vi "CPP-5168PuffReleaseAnalysisDevelopment.vi"() -> (5 "Plug in titles":string[](array[string]), 7 "Plug in values":string[](array[string]))   [LabVIEW 2012]
uses:
  Controls/Post_Process.ctl
  Globals/Meas_global.vi
  <vilib>/measure/mascope.llb/Transition Measurements 1 chan.vi
  <vilib>/Analysis/baseanly.llb/Quick Scale 1D.vi
  <vilib>/Analysis/baseanly.llb/Mean (DBL).vi
  <vilib>/measure/NI_MAPro.lvlib
  <vilib>/Analysis/NI_AALBase.lvlib
panel:
  in  "CPP-5168-FIDandPressure-Jan2013.vi Running Too?":bool=TRUE
  out "SampleLength":i32
  in  "MedianFilter(points)":i32=100
  in  "PufferCard":tag="PXI1Slot2"
  out "FFID1 2":cluster{dbl, dbl, dbl[]}[](graph)=[{3.0, 0.004, [20831.978051375965, 20830.73969787809, 20829.501417993935, 20828.26321171912, 20827.025079049276, 20825.787019980024, 20824.54903450699, 20823.311122625797, 20822.073284332073, 20820.83551962144, 20819.597828489525, 20818.360210931958, 20817.12266694436, 20815.885196522362, 20814.64779966159, 20813.410476357665, 20812.173226606224, 20810.936050402892, 20809.69894774329, 20808.461918623056, 20807.224963037814, 20805.98808098319, 20804.751272454818, 20803.51453744832, 20802.27787595934, 20801.041287983488, 20799.804773516407, 20798.56833255373, 20797.331965091074, 20796.09567112408, 20794.85945064838, 20793.623303659602, 20792.387230153374, 20791.151230125335, 20789.915303571113, 20788.679450486343, 20787.44367086665, 20786.20796470768, 20784.97233200505, 20783.736772754408, 20782.50128695138, 20781.265874591605, 20780.03053567071, 20778.795270184335, 20777.560078128114, 20776.32495949768, 20775.089914288666, 20773.854942496713, 20772.620044117455, 20771.38521914653, 20770.150467579566, 20768.915789412207, 20767.681184640092, 20766.44665325885, 20765.212195264125, 20763.977810651548, 20762.743499416763, 20761.509261555406, 20760.275097063113, 20759.041005935527, 20757.806988168282, 20756.573043757024, 20755.339172697382, 20754.105374985003, 20752.87165061553, 20751.637999584593, 20750.40442188784, 20749.17091752091, 20747.937486479444, 20746.704128759084, 20745.470844355466, 20744.237633264238, 20743.004495481044, 20741.771431001514, 20740.538439821306, 20739.30552193605, 20738.0726773414, 20736.839906032987, 20735.607208006462, 20734.37458325747, 20733.142031781652, 20731.909553574653, 20730.67714863212, 20729.444816949694, 20728.21255852302, 20726.980373347746, 20725.748261419518, 20724.516222733975, 20723.284257286774, 20722.052365073556, 20720.820546089963, 20719.588800331647, 20718.357127794257, 20717.125528473436, 20715.894002364836, 20714.662549464098, 20713.431169766878, 20712.19986326882, 20710.968629965573, 20709.737469852786, 20708.50638292611, 20707.27536918119, 20706.04442861368, 20704.81356121923, 20703.582766993495, 20702.35204593211, 20701.12139803074, 20699.890823285034, 20698.660321690637, 20697.429893243203, 20696.199537938388, 20694.96925577184, 20693.739046739214, 20692.50891083616, 20691.27884805833, 20690.04885840138, 20688.81894186096, 20687.58909843273, 20686.35932811234, 20685.12963089544, 20683.90000677769, 20682.670455754742, 20681.440977822254, 20680.211572975877, 20678.98224121127, 20677.75298252408, 20676.52379690998, 20675.29468436461, 20674.065644883634, 20672.836678462707, 20671.607785097483, 20670.378964783624, 20669.150217516788, 20667.921543292632, 20666.69294210681, 20665.464413954982, 20664.235958832807, 20663.007576735945, 20661.779267660055, 20660.551031600793, 20659.322868553823, 20658.094778514802, 20656.866761479392, 20655.63881744325, 20654.41094640204, 20653.183148351418, 20651.955423287054, 20650.727771204598, 20649.50019209972, 20648.272685968084, 20647.045252805343, 20645.817892607163, 20644.59060536921, 20643.363391087143, 20642.136249756626, 20640.90918137332, 20639.6821859329, 20638.455263431013, 20637.228413863337, 20636.001637225527, 20634.774933513254, 20633.548302722185, 20632.321744847977, 20631.095259886297, 20629.868847832815, 20628.642508683195, 20627.416242433108, 20626.19004907821, 20624.963928614176, 20623.737881036668, 20622.51190634136, 20621.286004523914, 20620.060175579998, 20618.83441950528, 20617.608736295435, 20616.383125946122, 20615.157588453014, 20613.93212381178, 20612.70673201809, 20611.481413067617, 20610.25616695602, 20609.03099367898, 20607.805893232162, 20606.58086561124, 20605.355910811882, 20604.131028829757, 20602.906219660545, 20601.681483299908, 20600.45681974352, 20599.232228987057, 20598.00771102619, 20596.78326585659, 20595.55889347393, 20594.33459387389, 20593.110367052133, 20591.886213004338, 20590.662131726178, 20589.438123213327, 20588.214187461464, 20586.990324466256, 20585.766534223385, 20584.54281672852, 20583.31917197734, 20582.095599965523, 20580.87210068874, 20579.648674142667, 20578.425320322985, 20577.202039225373, 20575.9788308455, 20574.75569517905, 20573.532632221697, 20572.309641969117, 20571.086724416993, 20569.863879561, 20568.64110739682, 20567.418407920126, 20566.195781126604, 20564.973227011928, 20563.750745571782, 20562.52833680184, 20561.306000697787, 20560.083737255303, 20558.861546470067, 20557.63942833776, 20556.417382854062, 20555.19541001466, 20553.97350981523, 20552.751682251455, 20551.52992731902, 20550.308245013606, 20549.086635330892, 20547.865098266564, 20546.643633816308, 20545.422241975804, 20544.200922740736, 20542.979676106785, 20541.758502069642, 20540.53740062499, 20539.31637176851, 20538.09541549589, 20536.87453180281, 20535.653720684964, 20534.43298213803, 20533.2123161577, 20531.991722739658, 20530.77120187959, 20529.55075357318, 20528.33037781612, 20527.110074604097, 20525.8898439328, 20524.66968579791, 20523.44960019512, 20522.229587120117, 20521.009646568586, 20519.789778536226, 20518.569983018715, 20517.35026001175, 20516.13060951102, 20514.91103151221, 20513.69152601101, 20512.472093003118, 20511.25273248422, 20510.033444450004, 20508.814228896164, 20507.595085818393, 20506.376015212383, 20505.15701707382, 20503.938091398402, 20502.71923818182, 20501.500457419766, 20500.281749107933, 20499.063113242017, 20497.844549817703, 20496.626058830694, 20495.407640276684, 20494.18929415136, 20492.971020450423, 20491.752819169564, 20490.534690304477, 20489.31663385086, 20488.09864980441, 20486.880738160817, 20485.662898915787, 20484.445132065004, 20483.227437604175, 20482.00981552899, 20480.792265835145, 20479.57478851835, 20478.357383574283, 20477.140050998656, 20475.922790787165, 20474.705602935504, 20473.488487439376, 20472.271444294474, 20471.054473496504, 20469.83757504116, 20468.620748924146, 20467.40399514116, 20466.187313687904, 20464.97070456007, 20463.75416775337, 20462.537703263497, 20461.321311086158, 20460.10499121705, 20458.888743651874, 20457.672568386337, 20456.456465416137, 20455.240434736974, 20454.024476344555, 20452.808590234585, 20451.592776402762, 20450.377034844794, 20449.161365556378, 20447.945768533224, 20446.73024377104, 20445.51479126552, 20444.29941101237, 20443.084103007306, 20441.86886724602, 20440.653703724227, 20439.43861243763, 20438.22359338193, 20437.008646552837, 20435.79377194606, 20434.578969557304, 20433.364239382274, 20432.14958141668, 20430.934995656226, 20429.720482096625, 20428.506040733584, 20427.291671562805, 20426.077374580003, 20424.863149780886, 20423.64899716116, 20422.434916716535, 20421.220908442723, 20420.00697233543, 20418.79310839037, 20417.579316603256, 20416.365596969794, 20415.15194948569, 20413.938374146666, 20412.724870948423, 20411.51143988668, 20410.298080957145, 20409.084794155533, 20407.871579477553, 20406.658436918922, 20405.44536647535, 20404.232368142548, 20403.019441916233, 20401.806587792114, 20400.59380576591, 20399.381095833338, 20398.168457990105, 20396.955892231927, 20395.74339855452, 20394.530976953603, 20393.318627424884, 20392.106349964088, 20390.894144566922, 20389.682011229102, 20388.469949946357, 20387.25796071439, 20386.04604352892, 20384.83419838567, 20383.622425280355, 20382.410724208694, 20381.1990951664, 20379.9875381492, 20378.776053152804, 20377.56464017293, 20376.353299205304, 20375.14203024564, 20373.93083328966, 20372.719708333087, 20371.508655371632, 20370.297674401023, 20369.086765416978, 20367.87592841522, 20366.665163391463, 20365.454470341436, 20364.243849260853, 20363.03330014545, 20361.82282299093, 20360.61241779303, 20359.402084547462, 20358.19182324996, 20356.981633896237, 20355.771516482022, 20354.56147100304, 20353.35149745501, 20352.141595833655, 20350.931766134705, 20349.72200835388, 20348.512322486906, 20347.302708529514, 20346.09316647742, 20344.883696326353, 20343.67429807204, 20342.464971710207, 20341.25571723658, 20340.046534646888, 20338.837423936853, 20337.62838510221, 20336.419418138674, 20335.21052304198, 20334.001699807857, 20332.792948432034, 20331.584268910236, 20330.37566123819, 20329.16712541163, 20327.958661426284, 20326.75026927788, 20325.541948962145, 20324.333700474814, 20323.125523811614, 20321.917418968278, 20320.709385940532, 20319.501424724112, 20318.293535314748, 20317.08571770817, 20315.87797190011, 20314.6702978863, 20313.46269566247, 20312.25516522436, 20311.047706567697, 20309.840319688214, 20308.63300458164, 20307.425761243718, 20306.218589670178, 20305.011489856748, 20303.80446179917, 20302.597505493177, 20301.3906209345, 20300.18380811888, 20298.977067042044, 20297.770397699736, 20296.56380008769, 20295.357274201633, 20294.150820037314, 20292.94443759046, 20291.738126856813, 20290.531887832112, 20289.325720512086, 20288.11962489248, 20286.913600969026, 20285.70764873747, 20284.50176819354, 20283.295959332983, 20282.09022215153, 20280.884556644934, 20279.678962808917, 20278.47344063923, 20277.26799013161, 20276.062611281795, 20274.857304085526, 20273.652068538548, 20272.446904636596, 20271.241812375414, 20270.036791750743, 20268.83184275832, 20267.626965393894, 20266.422159653204, 20265.217425531995, 20264.012763026003, 20262.80817213098, 20261.60365284266, 20260.399205156788, 20259.194829069114, 20257.990524575376, 20256.78629167132, 20255.582130352694, 20254.378040615233, 20253.174022454692, 20251.97007586681, 20250.766200847338, 20249.562397392012, 20248.358665496587, 20247.155005156805, 20245.951416368414, 20244.74789912716, 20243.54445342879, 20242.34107926905, 20241.13777664369, 20239.934545548454, 20238.731385979092, 20237.528297931352, 20236.325281400987, 20235.122336383734, 20233.919462875354, 20232.71666087159, 20231.51393036819, 20230.311271360908, 20229.108683845494, 20227.906167817695, 20226.703723273262, 20225.50135020795, 20224.299048617504, 20223.096818497677]}, ...(15 in all)]
  out "Valve":cluster{dbl, dbl, dbl[]}(graph)
  out "ValveShutAt":dbl format="%.2f"
  out "FFID2":T1(graph)
  out "Current Block No":i32
  out "FFID1":cluster{dbl, dbl, dbl[]}[](graph)
  out "SourceOffIndex":i32
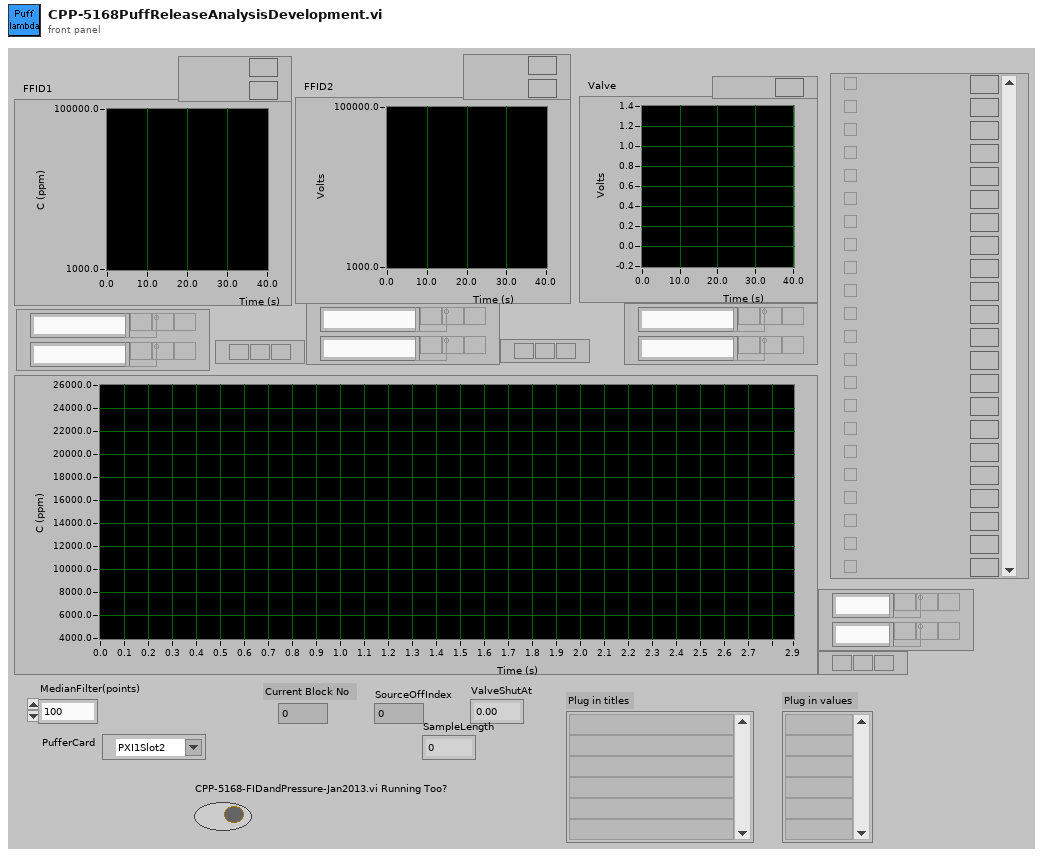
[diagram p1: front panel]
types:
  T1 = cluster{dbl, "SamplingRate":dbl, "Best Exponential Fit":dbl[]}[]
  T2 = typedef "Time_Trace_Cluster.ctl" = cluster{"Weighting":dbl[], "Time (s)":dbl[], "Voltage":dbl[], "Eng Values":dbl[]}
  T3 = typedef "Post_Process.ctl" = enum16{"Take New Data", "Post Process Raw Data File"}
  T4 = cluster{"start time":dbl, "end time":dbl, "ref levels":cluster{"high ref level":dbl, "mid ref level":dbl, "low ref level":dbl, "ref units":u16}}
  T5 = cluster{"x*y":dbl, "SamplingRate":dbl, "Filtered X":dbl[]}
  T6 = cluster{"x*y":dbl, "SamplingRate":dbl, "Filtered X":dbl[]}[]
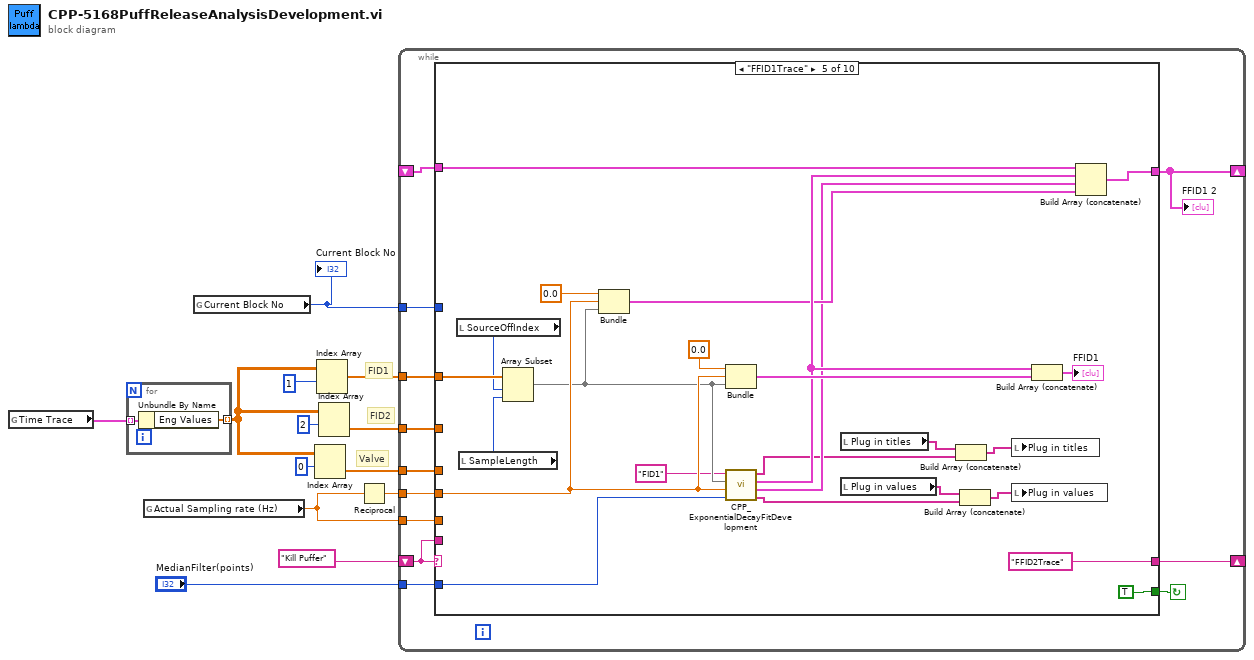
[diagram p0: block diagram]
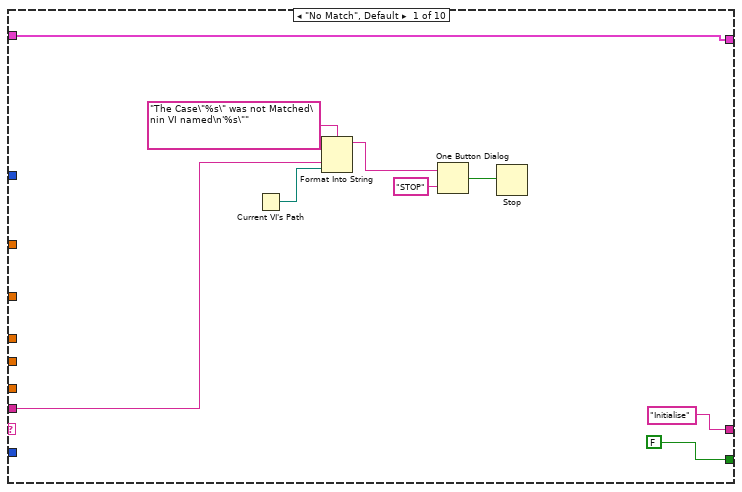
[diagram p2: hidden frame]
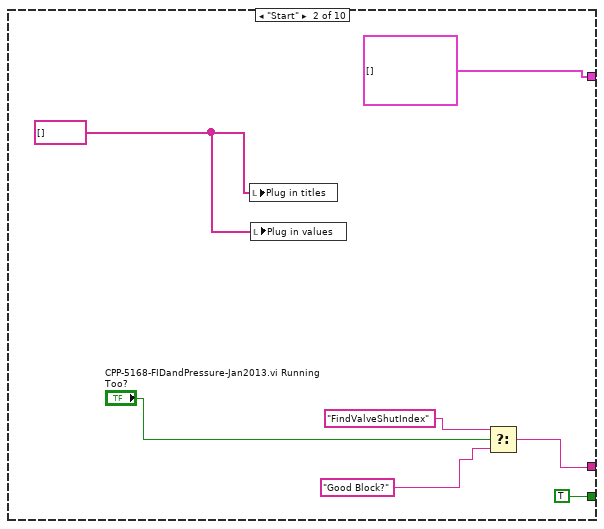
[diagram p3: hidden frame]
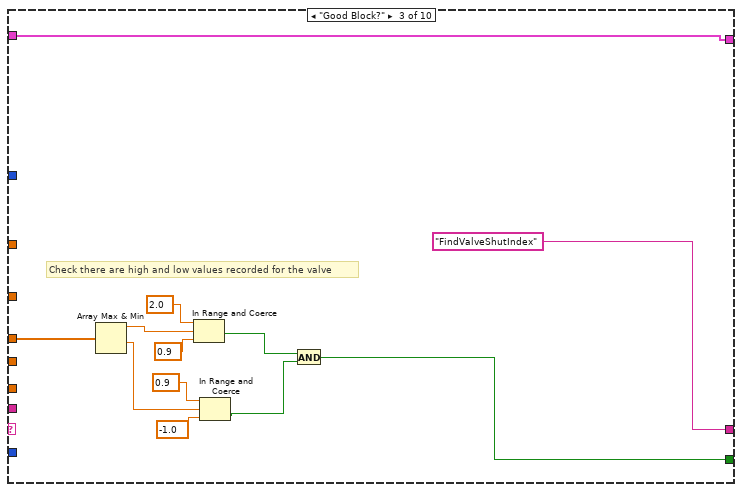
[diagram p4: hidden frame]
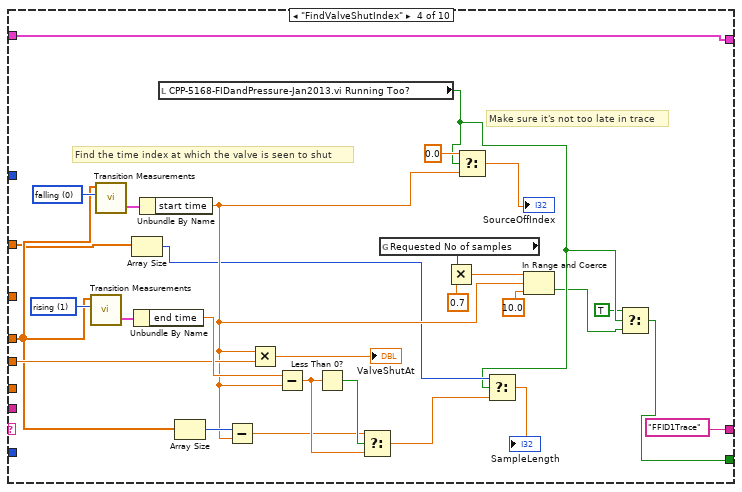
[diagram p5: hidden frame]
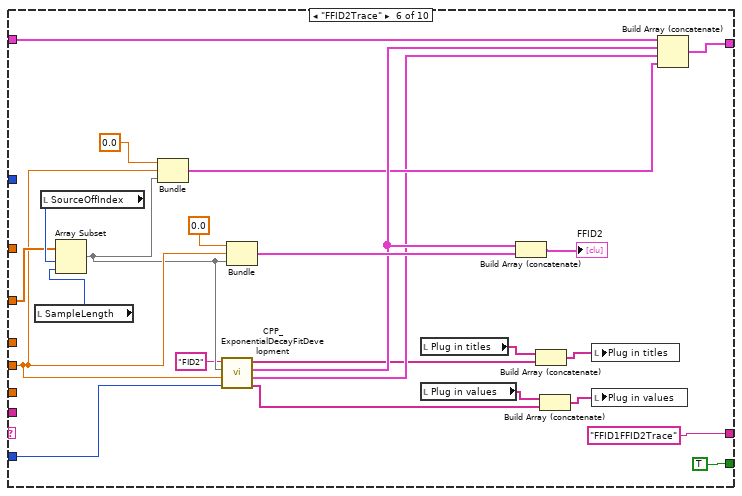
[diagram p6: hidden frame]
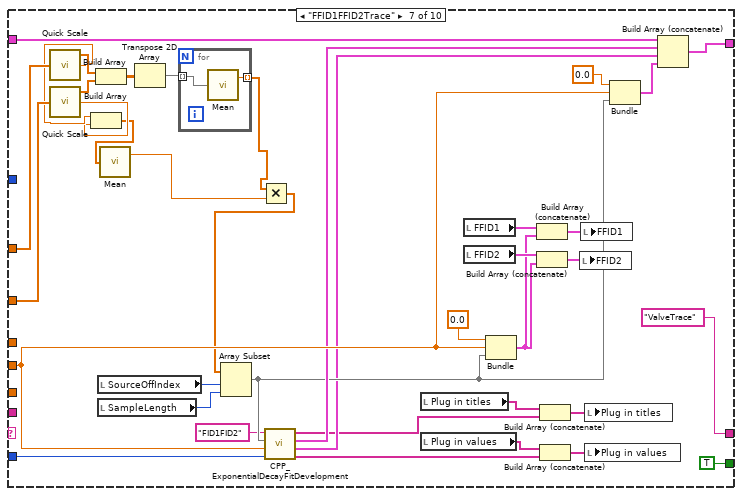
[diagram p7: hidden frame]
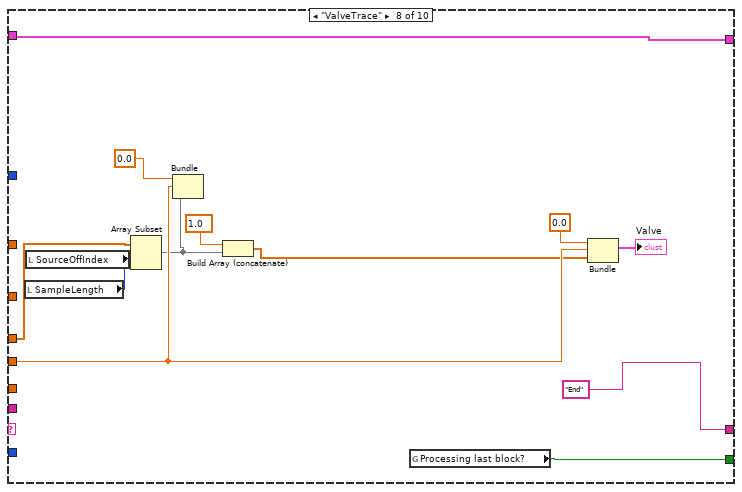
[diagram p8: hidden frame]
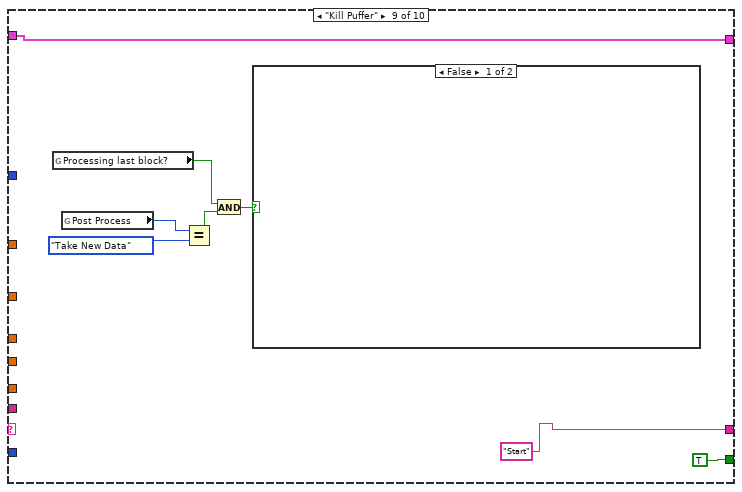
[diagram p9: hidden frame]
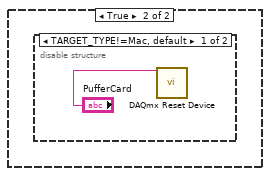
[diagram p10: hidden frame]
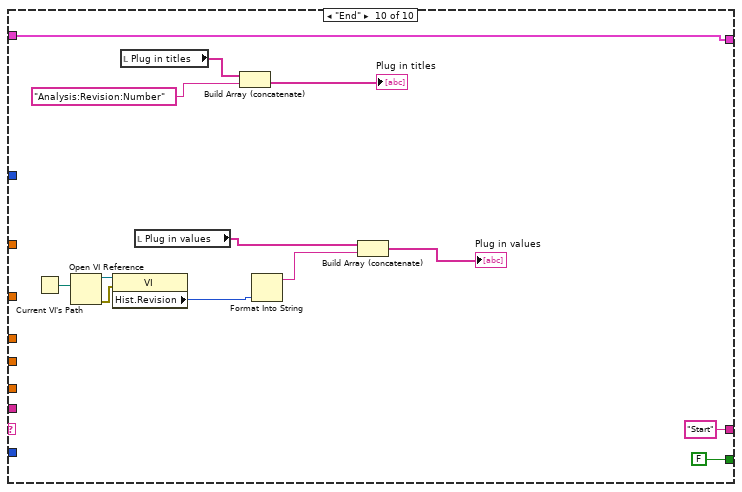
[diagram p12: hidden frame]
diagram:
  # "Valve"
  # "FID2"
  # "FID1"
  n1 = global read "Meas_global.vi" "Time Trace"() -> (w2:T2[])
  n2 = for {
    tunnel: w2 -> [w15] mode=indexing
    tunnel: [w14] -> w1 mode=indexing
    n3 = Unbundle By Name(w15) -> ("Eng Values"=w14:dbl[])
  }
  n4 = global read "Meas_global.vi" "Actual Sampling rate (Hz)"() -> (w5:dbl)
  n5 = global read "Meas_global.vi" "Current Block No"() -> (w10:i32)
  "Current Block No" <- w10
  n6 = Index Array(array=w1, index (row)=0) -> (element=w7:dbl[])  [unwired: 1 in]
  n7 = Index Array(array=w1, index (row)=1) -> (element=w11:dbl[])  [unwired: 1 in]
  n8 = Index Array(array=w1, index (row)=2) -> (element=w12:dbl[])  [unwired: 1 in]
  n9 = Reciprocal(x=w5) -> (1/x=w4:dbl)
  n10 = while {
    shift-left: "Kill Puffer" -> [w25]
    shift-right: [w26] -> _
    tunnel: w12 -> [w24]
    tunnel: w11 -> [w23]
    tunnel: w5 -> [w22]
    tunnel: w10 -> [w21]
    tunnel: w7 -> [w20]
    tunnel: w4 -> [w19]
    shift-right: [w17] -> _
    shift-left: _ -> [w18]
    tunnel: "MedianFilter(points)" -> [w16]
    stop <- w27 continue-if-true
    n11 = case shown="\"FFID1Trace\"" w25 {
      tunnel: [FALSE TRUE ("Processing last block?") w52 w57 TRUE ("Processing last block?") TRUE ("Processing last block?") TRUE ("Processing last block?") w177 TRUE ("Processing last block?") FALSE ("Processing last block?")] -> w27
      tunnel: ["Initialise" w37 "FindValveShutIndex" "FFID1Trace" "FFID2Trace" "FFID1FFID2Trace" "ValveTrace" "End" "Start" "Start" ("f")] -> w26
      tunnel: w25 -> [w31 _ _ _ _ _ _ _ _ _]
      tunnel: w24 -> [_ _ _ _ _ w128 w148 _ _ _]
      tunnel: w23 -> [_ _ _ w61 w106 _ w149 _ _ _]
      tunnel: w22 -> [_ _ _ _ _ _ _ _ _ _]
      tunnel: w21 -> [_ _ _ _ _ _ _ _ _ _]
      tunnel: w20 -> [_ _ w49 w69 _ _ _ w182 _ _]
      tunnel: w19 -> [_ _ _ w72 w99 w123 w163 w179 _ _]
      tunnel: [w28 cluster{dbl, dbl, dbl[]}[] [] w44 w77 w103 w127 w166 w173 w187 w205] -> w17
      tunnel: w18 -> [w28 _ w44 w77 w104 w126 w165 w173 w187 w205]
      tunnel: w16 -> [_ _ _ _ w94 w119 w160 _ _ _]
      frame "No Match", Default {
        n12 = Current VI's Path() -> (path=w30:path)
        n13 = Format Into String(format string="The Case\"%s\" was not Matched\nin VI named\n'%s\"" ("Format String"), w31, w30) -> (resulting string=w34:string)  [unwired: 2 in, 1 out]
        n14 = One Button Dialog(message=w34, button name ("OK")="STOP") -> (true=w32:bool)
        n15 = Stop(stop? (T)=w32) -> ()
      }
      frame "Start" {
        w41 = string[] []
        n16 = local write "Plug in titles"(w41) -> ()
        n17 = local write "Plug in values"(w41) -> ()
        n18 = Select(t="FindValveShutIndex", s="CPP-5168-FIDandPressure-Jan2013.vi Running Too?", f="Good Block?") -> (s? t:f=w37:string)
      }
      frame "Good Block?" {
        # "Check there are high and low values recorded for the valve"
        n19 = Array Max & Min(array=w49) -> (max value=w51:dbl, min value=w46:dbl)  [unwired: 2 out]
        n20 = In Range and Coerce(upper limit=2.0, x=w51, lower limit=0.9 ("y")) -> (In Range?=w53:bool)  [unwired: 1 out]
        n21 = In Range and Coerce(upper limit=0.9, x=w46, lower limit=-1.0 ("y")) -> (In Range?=w45:bool)  [unwired: 1 out]
        n22 = And(x=w53, y=w45) -> (x .and. y?=w52:bool)
      }
      frame "FindValveShutIndex" {
        w74 = u16 0 items=["falling", "rising"] ("polarity (rising)")
        w75 = u16 1 items=["falling", "rising"] ("polarity (rising)")
        # "Make sure it's not too late in trace"
        # "Find the time index at which the valve is seen to shut"
        n23 = call-poly <vilib>:"Transition Measurements.vi"("polarity (rising)"=w75, "signal in"=w69) -> ("measurement info"=w76:T4)  [unwired: 4 in, 5 out]
        n24 = call-poly <vilib>:"Transition Measurements.vi"("polarity (rising)"=w74, "signal in"=w69) -> ("measurement info"=w83:T4)  [unwired: 4 in, 5 out]
        n25 = Array Size(array=w61) -> (size(s)=w60:i32)
        n26 = Unbundle By Name(w76) -> ("end time"=w73:dbl)
        n27 = Unbundle By Name(w83) -> ("start time"=w66:dbl)
        n28 = local read "CPP-5168-FIDandPressure-Jan2013.vi Running Too?"() -> (w59:bool)
        n29 = Array Size(array=w69) -> (size(s)=w68:i32)
        n30 = Subtract(x=w68, y=w66) -> (x-y=w67:dbl)
        n31 = Multiply(x=w66, y=w72) -> (x*y=→"ValveShutAt":dbl)
        n32 = Subtract(x=w73, y=w66) -> (x-y=w70:dbl)
        n33 = Less Than 0?(x=w70) -> (x < 0?=w71:bool)
        n34 = Select(t=w67, s=w71, f=w70) -> (s? t:f=w63:dbl)
        n35 = global read "Meas_global.vi" "Requested No of samples"() -> (w82:i32)
        n36 = Multiply(x=w82, y=0.7 ("lower limit")) -> (x*y=w80:dbl)
        n37 = Select(t=0.0, s=w59, f=w66) -> (s? t:f=→"SourceOffIndex":dbl)
        n38 = Select(t=w60, s=w59, f=w63) -> (s? t:f=→"SampleLength":dbl)
        n39 = In Range and Coerce(upper limit=w80, x=w66, lower limit=10.0) -> (In Range?=w58:bool)  [unwired: 1 out]
        n40 = Select(t=TRUE, s=w59, f=w58) -> (s? t:f=w57:bool)
      }
      frame "FFID1Trace" {
        n41 = local read "SourceOffIndex"() -> (w105:i32)
        n42 = local read "SampleLength"() -> (w96:i32)
        n43 = Array Subset(array=w106, index=w105, length=w96) -> (w95:dbl[])
        n44 = Bundle(0.0, w99, w95) -> (w93:cluster{dbl, dbl, dbl[]})  [unwired: 1 out]
        n45 = Bundle(0.0, w99, w95) -> (w98:cluster{dbl, dbl, dbl[]})  [unwired: 1 out]
        n46 = call "CPP_ExponentialDecayFitDevelopment.vi"("MedianFilter(points)"=w94, "SamplingRate"=w99, "DecayData"=w95, "FID ID"="FID1") -> ("PlugInValues"=w85:string[], "smoothedCluster"=w92:T5, "GraphClusterArray"=w97:T1, "PlugInTitles"=w89:string[])
        n47 = local read "Plug in titles"() -> (w90:string[])
        n48 = local read "Plug in values"() -> (w86:string[])
        n49 = Build Array (concatenate)(w90, w89) -> (w88:string[])
        n50 = Build Array (concatenate)(w86, w85) -> (w87:string[])
        n51 = local write "Plug in titles"(w88) -> ()
        n52 = local write "Plug in values"(w87) -> ()
        n53 = Build Array (concatenate)(w97, w98) -> (→"FFID1":T1)
        n54 = Build Array (concatenate)(w104, w97, w92, w93) -> (w103:T6)
      }
      frame "FFID2Trace" {
        n55 = local read "SampleLength"() -> (w120:i32)
        n56 = local read "SourceOffIndex"() -> (w130:i32)
        n57 = Array Subset(array=w128, index=w130, length=w120) -> (w118:dbl[])
        n58 = Bundle(0.0, w123, w118) -> (w117:cluster{dbl, dbl, dbl[]})  [unwired: 1 out]
        n59 = call "CPP_ExponentialDecayFitDevelopment.vi"("MedianFilter(points)"=w119, "SamplingRate"=w123, "DecayData"=w118, "FID ID"="FID2") -> ("PlugInValues"=w109:string[], "smoothedCluster"=w116:T5, "GraphClusterArray"=w121:T1, "PlugInTitles"=w110:string[])
        n60 = Bundle(0.0, w123, w118) -> (w122:cluster{dbl, dbl, dbl[]})  [unwired: 1 out]
        n61 = local read "Plug in titles"() -> (w114:string[])
        n62 = local read "Plug in values"() -> (w111:string[])
        n63 = Build Array (concatenate)(w121, w122) -> (→"FFID2":T1)
        n64 = Build Array (concatenate)(w114, w110) -> (w113:string[])
        n65 = Build Array (concatenate)(w111, w109) -> (w112:string[])
        n66 = local write "Plug in titles"(w113) -> ()
        n67 = local write "Plug in values"(w112) -> ()
        n68 = Build Array (concatenate)(w126, w121, w116, w117) -> (w127:T6)
      }
      frame "FFID1FFID2Trace" {
        n69 = call-poly <vilib>:"Quick Scale.vi"("X"=w149) -> ("Y[i]=X[i]/Max|X|"=w147:dbl[], "max|X|"=w136:dbl)  [unwired: 1 out]
        n70 = call-poly <vilib>:"Quick Scale.vi"("X"=w148) -> ("Y[i]=X[i]/Max|X|"=w146:dbl[], "max|X|"=w135:dbl)  [unwired: 1 out]
        n71 = Build Array(w136, w135) -> (w134:dbl[])
        n72 = Build Array(w147, w146) -> (w140:dbl[][])
        n73 = local read "SourceOffIndex"() -> (w168:i32)
        n74 = local read "SampleLength"() -> (w161:i32)
        n75 = call-poly <vilib>:"Mean.vi"("X"=w134) -> ("mean"=w133:dbl)  [unwired: 1 out]
        n76 = Transpose 2D Array(2D array=w140) -> (transposed array=w139:dbl[][])
        n77 = for {
          tunnel: w139 -> [w172] mode=indexing
          tunnel: [w171] -> w137 mode=indexing
          n78 = call-poly <vilib>:"Mean.vi"("X"=w172) -> ("mean"=w171:dbl)  [unwired: 1 out]
        }
        n79 = Multiply(x=w137, y=w133) -> (x*y=w138:dbl[])
        n80 = Array Subset(array=w138, index=w168, length=w161) -> (w159:dbl[])
        n81 = call "CPP_ExponentialDecayFitDevelopment.vi"("MedianFilter(points)"=w160, "SamplingRate"=w163, "DecayData"=w159, "FID ID"="FID1FID2") -> ("PlugInValues"=w150:string[], "smoothedCluster"=w157:T5, "GraphClusterArray"=w162:T1, "PlugInTitles"=w151:string[])
        n82 = local read "Plug in titles"() -> (w155:string[])
        n83 = local read "Plug in values"() -> (w152:string[])
        n84 = local read "FFID1"() -> (w145:cluster{dbl, dbl, dbl[]}[])
        n85 = local read "FFID2"() -> (w144:T1)
        n86 = Bundle(0.0, w163, w159) -> (w142:cluster{dbl, dbl, dbl[]})  [unwired: 1 out]
        n87 = Build Array (concatenate)(w145, w142) -> (w141:cluster{dbl, dbl, dbl[]}[])
        n88 = Build Array (concatenate)(w144, w142) -> (w143:T1)
        n89 = Build Array (concatenate)(w155, w151) -> (w154:string[])
        n90 = Build Array (concatenate)(w152, w150) -> (w153:string[])
        n91 = local write "FFID2"(w143) -> ()
        n92 = local write "FFID1"(w141) -> ()
        n93 = local write "Plug in titles"(w154) -> ()
        n94 = local write "Plug in values"(w153) -> ()
        n95 = Bundle(0.0, w163, w159) -> (w158:cluster{dbl, dbl, dbl[]})  [unwired: 1 out]
        n96 = Build Array (concatenate)(w165, w162, w157, w158) -> (w166:T6)
      }
      frame "ValveTrace" {
        n97 = local read "SampleLength"() -> (w175:i32)
        n98 = local read "SourceOffIndex"() -> (w184:i32)
        n99 = Array Subset(array=w182, index=w184, length=w175) -> (w178:dbl[])
        n100 = Bundle(0.0, w179, w178) -> ()  [unwired: 2 out]
        n101 = Build Array (concatenate)(1.0, w178) -> (w174:dbl[])
        n102 = global read "Meas_global.vi" "Processing last block?"() -> (w177:bool)
        n103 = Bundle(0.0, w179, w174) -> (→"Valve":cluster{dbl, dbl, dbl[]})  [unwired: 1 out]
      }
      frame "Kill Puffer" {
        n104 = global read "Meas_global.vi" "Processing last block?"() -> (w190:bool)
        n105 = global read "Meas_global.vi" "Post Process"() -> (w192:T3)
        n106 = Equal?(x=w192, y=Post_Process."Take New Data" ("Post Process")) -> (x = y?=w189:bool)
        n107 = And(x=w190, y=w189) -> (x .and. y?=w188:bool)
        n108 = case shown="False" w188 {
          frame False {
          }
          frame True {
            n109 = disable-structure shown="TARGET_TYPE!=Mac, default" {
              frame condition #0 (active) {
                n110 = call <vilib>:"DAQmx Reset Device.vi"("device in"="PufferCard") -> ()  [unwired: 14 in, 1 out]
              }
              frame condition #1 {
              }
            }
          }
        }
      }
      frame "End" {
        n111 = Current VI's Path() -> (path=w203:path)
        n112 = Open VI Reference(vi path=w203) -> (vi reference=w202:refnum<vi>, error out=w201:errorcluster)  [unwired: 5 in]
        n113 = property class="VI"(reference=w202, error in=w201) -> ("Hist.Revision"=w200:u32)  [unwired: 2 out]
        n114 = local read "Plug in titles"() -> (w199:string[])
        n115 = local read "Plug in values"() -> (w196:string[])
        n116 = Build Array (concatenate)(w199, "Analysis:Revision:Number") -> (→"Plug in titles":string[])
        n117 = Format Into String(w200) -> (resulting string=w195:string)  [unwired: 3 in, 1 out]
        n118 = Build Array (concatenate)(w196, w195) -> (→"Plug in values":string[])
      }
    }
    "FFID1 2" <- w17
  }
